vi "GOOP_LVClass_Provider_OnCommand.vi"(10 "Command Tag":string, 11 "objects":T1[](array[typedef])) -> ()   [LabVIEW 2020]
uses:
  <resource>/Framework/Providers/API/ItemRef.ctl
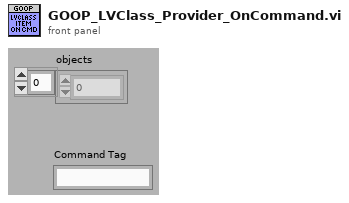
[diagram p1: front panel]
types:
  T1 = typedef "ItemRef.ctl" = u64
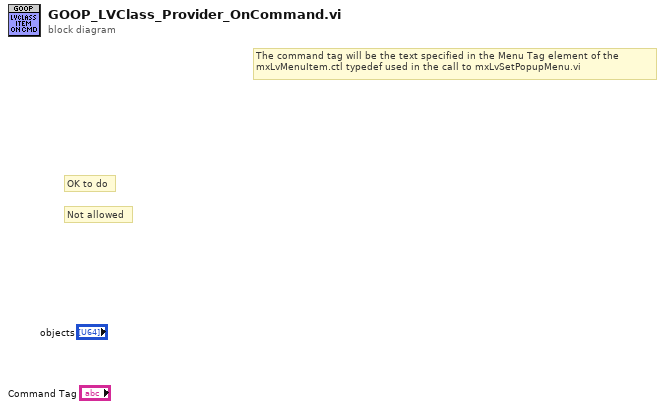
[diagram p0: block diagram]
diagram:
  # "Not allowed"
  # "OK to do"
  # "The command tag will be the text specified in the Menu Tag element of the \nmxLvMenuItem.ctl typedef used in the call to mxLvSetPopupMenu.vi"
